vi "TagBus_Write Table from Cluster.vi"(7 "Clust Refnum":refnum<vi>, 10 "Index Array":i32[](array[numeric]), 11 "TagBus in":refnum<class "TagBus.lvclass">) -> (3 "TagBus out":refnum<class "TagBus.lvclass">)   [LabVIEW 2015, in "TagBus.lvclass"]
uses:
  TagBus.lvclass
  TagBus.lvclass/TagBus.ctl
  <vilib>/NI/Tag Bus/table/data polymorphs/write one/write Single.vi
  <vilib>/NI/Tag Bus/table/data polymorphs/write one/write I64.vi
  <vilib>/NI/Tag Bus/table/data polymorphs/write one/write I32.vi
  <vilib>/NI/Tag Bus/table/data polymorphs/write one/write I16.vi
  <vilib>/NI/Tag Bus/table/data polymorphs/write one/write I8.vi
  <vilib>/NI/Tag Bus/table/data polymorphs/write one/write U64.vi
  <vilib>/NI/Tag Bus/table/data polymorphs/write one/write U32.vi
  <vilib>/NI/Tag Bus/table/data polymorphs/write one/write U16.vi
  <vilib>/NI/Tag Bus/table/data polymorphs/write one/write U8.vi
  <vilib>/NI/Tag Bus/table/data polymorphs/write one/write Boolean.vi
  <vilib>/NI/Tag Bus/table/data polymorphs/write one/write String.vi
  <vilib>/NI/Tag Bus/table/data polymorphs/write one/write Double.vi
  <vilib>/NI/Tag Bus/table/data table.lvlib
  <vilib>/Utility/Data Type/NI_Data Type.lvlib
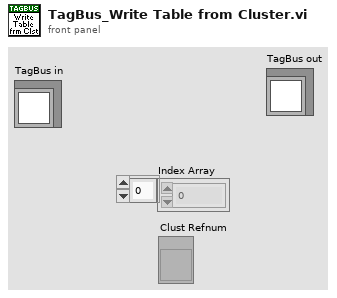
[diagram p1: front panel]
types:
  T1 = typedef "tag bus.lvlib/data table.lvlib/data table.ctl" = cluster{"Double":dbl[], "Single":sgl[], "I64":i64[], "I32":i32[], "I16":i16[], "I8":i8[], "U64":u64[], "U32":u32[], "U16":u16[], "U8":u8[], "Boolean":bool[], "String":string[], "Array of Double":cluster{"DBL Array":dbl[]}[], "Array of Single":cluster{"SGL Array":sgl[]}[], "Array of I64":cluster{"I64 Array":i64[]}[], "Array of I32":cluster{"I32 Array":i32[]}[], "Array of I16":cluster{"I16 Array":i16[]}[], "Array of I8":cluster{"I8 Array":i8[]}[], "Array of U64":cluster{"U64 Array":u64[]}[], "Array of U32":cluster{"U32 Array":u32[]}[], "Array of U16":cluster{"U16 Array":u16[]}[], "Array of U8":cluster{"U8 Array":u8[]}[], "Array of Boolean":cluster{"Boolean Array":bool[]}[], "Array of String":cluster{"String Array":string[]}[]}
  T2 = typedef "NI_Data Type.lvlib/Data Type.ctl" = enum8{"Invalid Type", "Void", "I8", "I16", "I32", "I64", "U8", "U16", "U32", "U64", "Single Float", "Double Float", "Extended Float", "Single Complex", "Double Complex", "Extended Complex", "Enum U8", "Enum U16", "Enum U32", "Enum U64", "Single Float With Unit", "Double Float With Unit", "Extended Float With Unit", "Single Complex with Unit", "Double Complex with Unit", "Extended Complex with Unit", "Boolean", "String", "Path", "Picture", "Tag", "Array", "Cluster", "Variant", "LV Variant", "Waveform", "Timestamp", "Digital Waveform", "Digital Data", "ExpressData", "Refnum", "External Data", "VI", "Poly VI", "LabVIEW Class Instance", "Fixed Point"}
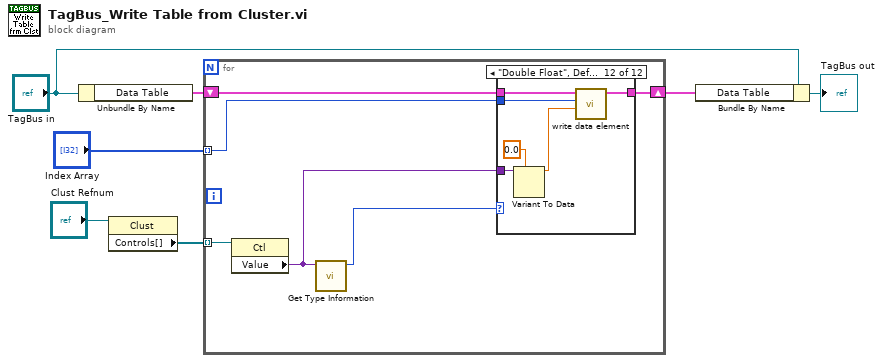
[diagram p0: block diagram]
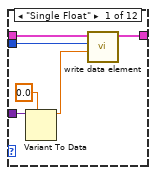
[diagram p2: hidden frame]
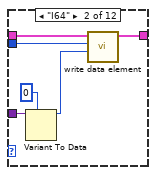
[diagram p3: hidden frame]
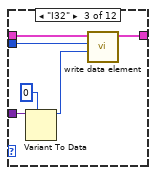
[diagram p4: hidden frame]
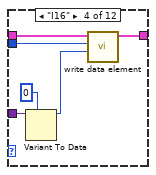
[diagram p5: hidden frame]
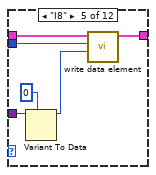
[diagram p6: hidden frame]
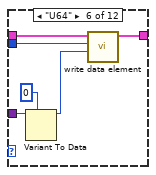
[diagram p7: hidden frame]
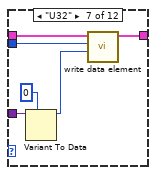
[diagram p8: hidden frame]
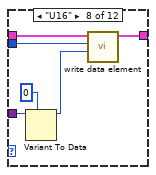
[diagram p9: hidden frame]
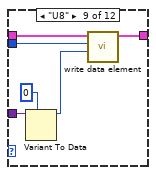
[diagram p10: hidden frame]
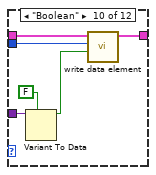
[diagram p11: hidden frame]
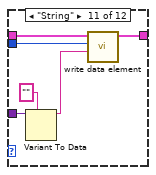
[diagram p12: hidden frame]
diagram:
  n1 = Unbundle By Name("TagBus in") -> ("Data Table"=w6:T1)
  n2 = property class="Clust"(reference="Clust Refnum") -> ("Controls[]"=w1:refnum<vi>[])  [unwired: 1 in, 2 out]
  n3 = for {
    tunnel: "Index Array" -> [w11] mode=indexing
    shift-right: [w12] -> w4
    shift-left: w6 -> [w13]
    tunnel: w1 -> [w10] mode=indexing
    n4 = property class="Ctl"(reference=w10) -> ("Value"=w9:variant)  [unwired: 1 in, 2 out]
    n5 = call <vilib>:"Get Type Information.vi"("Variant"=w9) -> ("Type"=w8:T2)  [unwired: 6 in, 4 out]
    n6 = case shown="\"Double Float\", Default" w8 {
      tunnel: w13 -> [w19 w25 w31 w37 w43 w49 w55 w61 w67 w73 w79 w85]
      tunnel: [w18 w24 w30 w36 w42 w48 w54 w60 w66 w72 w78 w84] -> w12
      tunnel: w11 -> [w17 w23 w29 w35 w41 w47 w53 w59 w65 w71 w77 w83]
      tunnel: w9 -> [w16 w22 w28 w34 w40 w46 w52 w58 w64 w70 w76 w82]
      frame "Single Float" {
        n7 = Variant To Data(type=sgl 0.0, Variant=w16) -> (data=w14:sgl)  [unwired: 1 in, 1 out]
        n8 = call-poly <vilib>:"write data element.vi"("value"=w14, "index"=w17, "data table in"=w19) -> ("data table out"=w18:T1)  [unwired: 8 in]
      }
      frame "I64" {
        n9 = Variant To Data(type=i64 0, Variant=w22) -> (data=w20:i64)  [unwired: 1 in, 1 out]
        n10 = call-poly <vilib>:"write data element.vi"("value"=w20, "index"=w23, "data table in"=w25) -> ("data table out"=w24:T1)  [unwired: 8 in]
      }
      frame "I32" {
        n11 = Variant To Data(type=0, Variant=w28) -> (data=w26:i32)  [unwired: 1 in, 1 out]
        n12 = call-poly <vilib>:"write data element.vi"("value"=w26, "index"=w29, "data table in"=w31) -> ("data table out"=w30:T1)  [unwired: 8 in]
      }
      frame "I16" {
        n13 = Variant To Data(type=i16 0, Variant=w34) -> (data=w32:i16)  [unwired: 1 in, 1 out]
        n14 = call-poly <vilib>:"write data element.vi"("value"=w32, "index"=w35, "data table in"=w37) -> ("data table out"=w36:T1)  [unwired: 8 in]
      }
      frame "I8" {
        n15 = Variant To Data(type=i8 0, Variant=w40) -> (data=w38:i8)  [unwired: 1 in, 1 out]
        n16 = call-poly <vilib>:"write data element.vi"("value"=w38, "index"=w41, "data table in"=w43) -> ("data table out"=w42:T1)  [unwired: 8 in]
      }
      frame "U64" {
        n17 = Variant To Data(type=u64 0, Variant=w46) -> (data=w44:u64)  [unwired: 1 in, 1 out]
        n18 = call-poly <vilib>:"write data element.vi"("value"=w44, "index"=w47, "data table in"=w49) -> ("data table out"=w48:T1)  [unwired: 8 in]
      }
      frame "U32" {
        n19 = Variant To Data(type=u32 0, Variant=w52) -> (data=w50:u32)  [unwired: 1 in, 1 out]
        n20 = call-poly <vilib>:"write data element.vi"("value"=w50, "index"=w53, "data table in"=w55) -> ("data table out"=w54:T1)  [unwired: 8 in]
      }
      frame "U16" {
        n21 = Variant To Data(type=u16 0, Variant=w58) -> (data=w56:u16)  [unwired: 1 in, 1 out]
        n22 = call-poly <vilib>:"write data element.vi"("value"=w56, "index"=w59, "data table in"=w61) -> ("data table out"=w60:T1)  [unwired: 8 in]
      }
      frame "U8" {
        n23 = Variant To Data(type=u8 0, Variant=w64) -> (data=w62:u8)  [unwired: 1 in, 1 out]
        n24 = call-poly <vilib>:"write data element.vi"("value"=w62, "index"=w65, "data table in"=w67) -> ("data table out"=w66:T1)  [unwired: 8 in]
      }
      frame "Boolean" {
        n25 = Variant To Data(type=FALSE, Variant=w70) -> (data=w68:bool)  [unwired: 1 in, 1 out]
        n26 = call-poly <vilib>:"write data element.vi"("value"=w68, "index"=w71, "data table in"=w73) -> ("data table out"=w72:T1)  [unwired: 8 in]
      }
      frame "String" {
        n27 = Variant To Data(type="", Variant=w76) -> (data=w74:string)  [unwired: 1 in, 1 out]
        n28 = call-poly <vilib>:"write data element.vi"("value"=w74, "index"=w77, "data table in"=w79) -> ("data table out"=w78:T1)  [unwired: 8 in]
      }
      frame "Double Float", Default {
        n29 = Variant To Data(type=0.0, Variant=w82) -> (data=w80:dbl)  [unwired: 1 in, 1 out]
        n30 = call-poly <vilib>:"write data element.vi"("value"=w80, "index"=w83, "data table in"=w85) -> ("data table out"=w84:T1)  [unwired: 8 in]
      }
    }
  }
  n31 = Bundle By Name(cluster="TagBus in", "Data Table"=w4) -> (→"TagBus out":refnum<class "TagBus.lvclass">)
